vi "WriteFile.vi"(8 "error in (no error)":errorcluster, 10 "data":i32[](array[numeric]), 11 "RWFile in":refnum<class "RWFile.lvclass">) -> (0 "error out":errorcluster, 3 "RWFile out":refnum<class "RWFile.lvclass">)   [LabVIEW 2021, in "RWFile.lvclass"]
uses:
  RWFile.lvclass
  RWFile.lvclass/RWFile.ctl
  File/File.lvclass
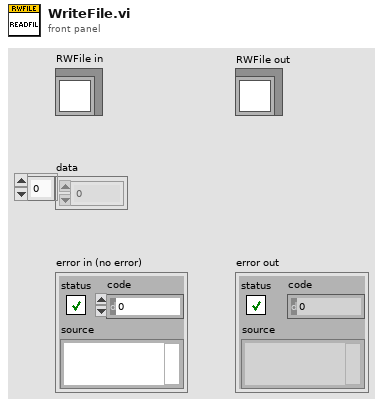
[diagram p1: front panel]
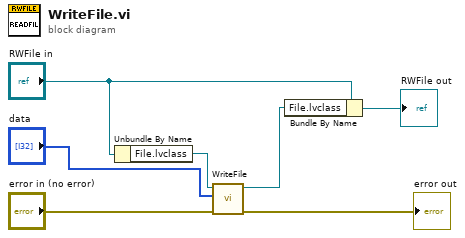
[diagram p0: block diagram]
diagram:
  n1 = Unbundle By Name("RWFile in") -> ("File.lvclass"=w5:refnum<class "File.lvclass">)
  n2 = call "WriteFile.vi"("error in (no error)"="error in (no error)", "data"="data", "File in"=w5) -> ("error out"=→"error out":errorcluster, "File out"=w1:refnum<class "File.lvclass">)  [unwired: 7 in]
  n3 = Bundle By Name(cluster="RWFile in", "File.lvclass"=w1) -> (→"RWFile out":refnum<class "RWFile.lvclass">)
